vi "Load.vi"(8 "error in":errorcluster, 10 "Source":string, 11 "PCAN Basic Base Configure Strategy in":refnum<class "PCAN Basic Base Configure Strategy.lvclass">) -> (0 "error out":errorcluster, 3 "PCAN Basic Base Configure Strategy out":refnum<class "PCAN Basic Base Configure Strategy.lvclass">)   [LabVIEW 2025, in "PCAN Basic Base Configure Strategy.lvclass"]
uses:
  PCAN Basic Base Configure Strategy.lvclass
  Source/Interfaces/IConfiguration/IConfiguration.lvclass
  Source/Config from JSON/Config from JSON.lvclass
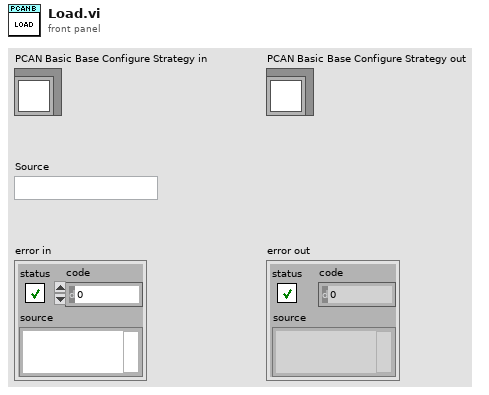
[diagram p1: front panel]
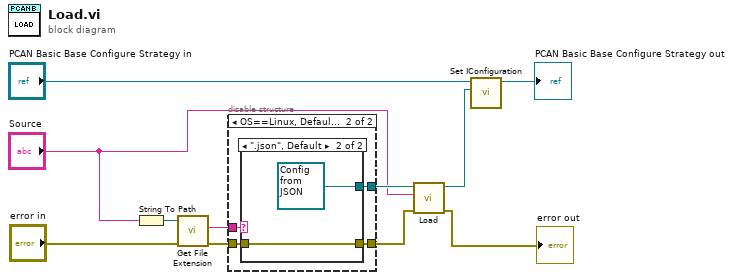
[diagram p0: block diagram]
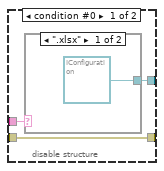
[diagram p2: hidden frame]
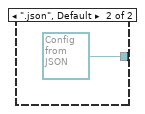
[diagram p3: hidden frame]
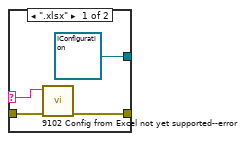
[diagram p4: hidden frame]
diagram:
  n1 = String To Path(string="Source") -> (path=w10:path)
  n2 = call <vilib>:"Get File Extension.vi"("error in (no error)"="error in", "file"=w10) -> ("error out"=w2:errorcluster, "lowercase file extension"=w9:string)  [unwired: 5 in, 3 out]
  n3 = disable-structure shown="OS==Linux, Default" {
    disable-tunnel: w9 -> [w14 w17]
    disable-tunnel: [w13 w20] -> w8
    disable-tunnel: w2 -> [w12 w19]
    disable-tunnel: [w12 w18] -> w1
    frame condition #0 {
      n4 = case shown="\".xlsx\"" w14 {
        tunnel: [refnum<class "IConfiguration.lvclass"> refnum ("IConfiguration.lvclass") refnum<class "Config from JSON.lvclass"> refnum ("Config from JSON.lvclass")] -> w13
        frame ".xlsx" {
        }
        frame ".json", Default {
        }
      }
    }
    frame condition #1 (active) {
      n5 = case shown="\".json\", Default" w17 {
        selector: w17 -> [w22 _]
        tunnel: [refnum<class "IConfiguration.lvclass"> refnum ("IConfiguration.lvclass") refnum<class "Config from JSON.lvclass"> refnum ("Config from JSON.lvclass")] -> w20
        tunnel: w19 -> [w24 w25]
        tunnel: [w23 w25] -> w18
        frame ".xlsx" {
          n6 = call "9102 Config from Excel not yet supported--error.vi"("error in"=w24, "Argument"=w22) -> ("error out"=w23:errorcluster)  [unwired: 8 in, 1 out]
        }
        frame ".json", Default {
        }
      }
    }
  }
  n7 = call-dynamic "Load.vi"("error in"=w1, "Source"="Source", "IConfiguration in"=w8) -> ("error out"=→"error out":errorcluster, "IConfiguration out"=w11:refnum<class "IConfiguration.lvclass">)  [unwired: 7 in]
  n8 = call-dynamic "Set IConfiguration.vi"("IConfiguration"=w11, "PCAN Basic in"="PCAN Basic Base Configure Strategy in") -> ("PCAN Basic out"=→"PCAN Basic Base Configure Strategy out":refnum<class "PCAN Basic Base Configure Strategy.lvclass">)  [unwired: 9 in]
